vi "General wait for movement to stop.vi"(0 "System no.":i32=1, 2 "Axes to wait for":string[](array[string]), 3 "All axes?":bool=TRUE, 4 "Additional wait time, ms":u32, 5 "error in":errorcluster, 6 "Add. wait only?":bool, 7 "Polling cycle \ntime, ms":u32=10, 12 "Stop refnum":refnum<vi>) -> (14 "Stopped":bool, 19 "error out":errorcluster)   [LabVIEW 2026]
doc: "This VI waits for the specified axes to stop. An additional wait time can be specified. The wait method depends on the system to command. PI_GCS2_Configuration_Setup.vi must be run before running this VI. If Add. wait only? is TRUE, VI waits the given Additional wait time only. Requires Wait for axes to stop.vi, #5.vi, STA?.vi, #5_old.vi, ONT?.vi and Wait for hexapod system axes to stop.vi to be present. VI does not time out, so when using as a sub-VI, use Stop refnum to stop VI from caller.\n\nAnalog: If VOL was commanded or velocity control mode (VCO) is OFF, Add. wait only? must be TRUE, otherwise FALSE.\nE-816: All axes? = FALSE. only one axis per command allowed.\nC-887, F-206, M-8X0: For GCS syntax version = GCS 1.0 (Check with CSV?.vi. If CSV?.vi is not supported, syntax version is GCS 1.0), VI will not wait for INI procedure to complete."
uses:
  Communication/Syntax.ctl
  GeneralCommands/Global2 (Array).vi
  AnalogControl/Global Analog.vi
  Communication/Global1.vi
panel:
  in  "Local stop":bool
  # "This vi waits for the specified axes to stop. An additional wait\ntime can be specified. The wait method depends on the system\nto command. If \"Add. wait only?\" is TRUE, VI waits the given \nadditional wait time only. \"XXX_Configuration_Setup.vi\" must be\nrun before running this vi."
  # "Wait for"
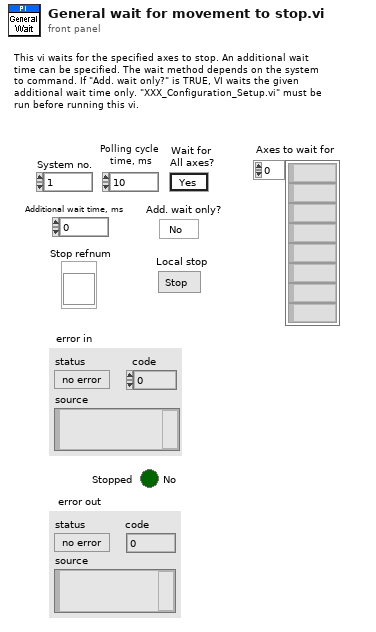
[diagram p1: front panel]
types:
  T1 = typedef "Controller names.ctl" = enum16{"None", "Analog", "C-702", "C-413", "C-414", "C-843", "C-843.PM", "C-844", "C-848", "C-865", "C-866", "C-867", "C-877", "C-880", "C-884", "C-885", "C-886", "C-887", "C-891", "E-135", "E-516", "E-517", "E-518", "E-709", "E-710", "E-712", "E-725", "E-727", "E-753", "E-754", "E-755", "E-761", "E-816", "E-861", "E-870", "E-871", "E-872", "E-873", "E-874", "F-206", "HydraPollux", "M-840", "M-850", "M-8X0", "Mercury", "Mercury_GCS", "PI_GCS2"}
  T2 = cluster{"Conn. axes":string[], "Controller name":T1}[]
  T3 = cluster{"Conn. axes":string[], "Controller name":T1}
  T4 = typedef "Syntax.ctl" = enum16{"GCS 1.0", "GCS 2.0", "GCS 3.0"}
  T5 = cluster{"Conversion factor":dbl[], "Velocity":dbl[], "Velocity control mode":bool, "AO.Resolution":dbl, "Lower voltage limit (V)":dbl, "Upper voltage limit (V)":dbl, "AO_WF_T (s)":dbl, "AI Sample Rate":dbl, "AI Samples/Channel":i32, "Hyperbit":bool, "Offset (V)":dbl[], "Hyperbit StayOnPos":bool, "Gain (V)":dbl[], "Bit rate (Hz)":dbl, "PWM rate (Hz)":dbl, "HyperBit Password":string, "AO.MaxRate":dbl, "Conversion offset":dbl[]}[]
  T6 = cluster{"Conversion factor":dbl[], "Velocity":dbl[], "Velocity control mode":bool, "AO.Resolution":dbl, "Lower voltage limit (V)":dbl, "Upper voltage limit (V)":dbl, "AO_WF_T (s)":dbl, "AI Sample Rate":dbl, "AI Samples/Channel":i32, "Hyperbit":bool, "Offset (V)":dbl[], "Hyperbit StayOnPos":bool, "Gain (V)":dbl[], "Bit rate (Hz)":dbl, "PWM rate (Hz)":dbl, "HyperBit Password":string, "AO.MaxRate":dbl, "Conversion offset":dbl[]}
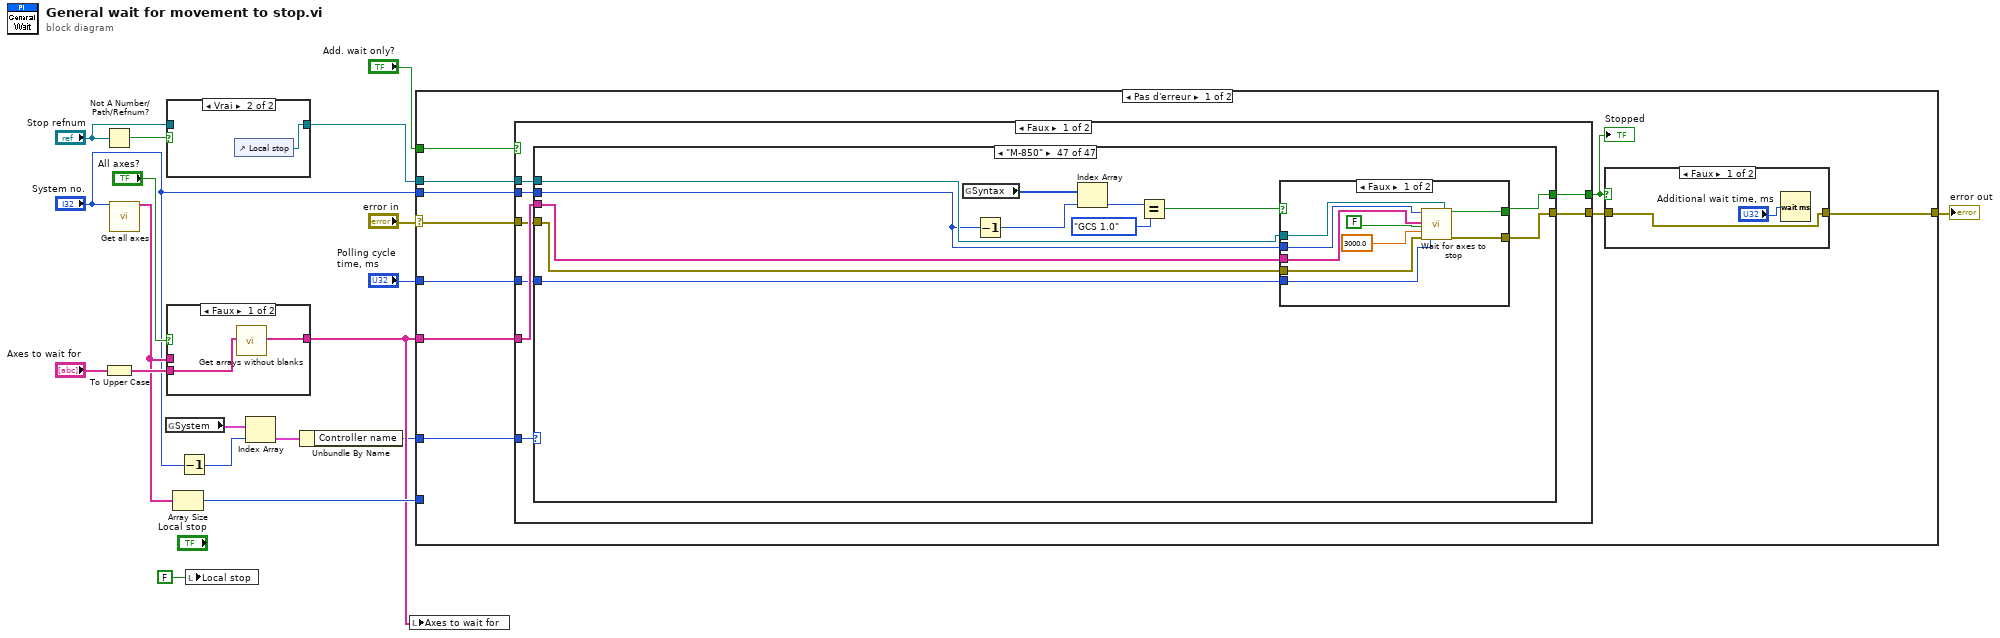
[diagram p0: block diagram]
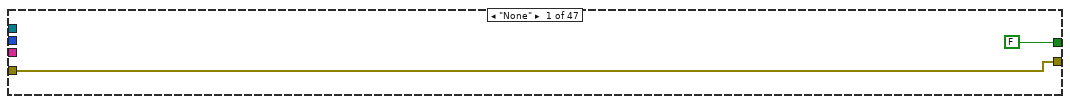
[diagram p4: hidden frame]
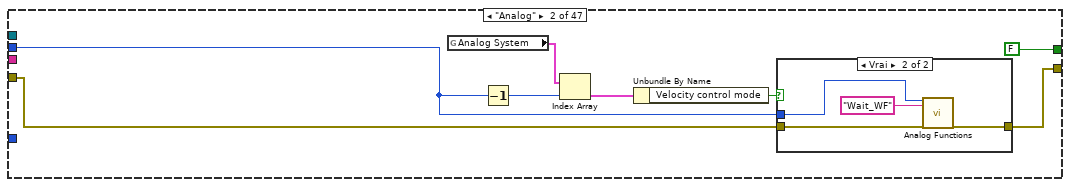
[diagram p5: hidden frame]
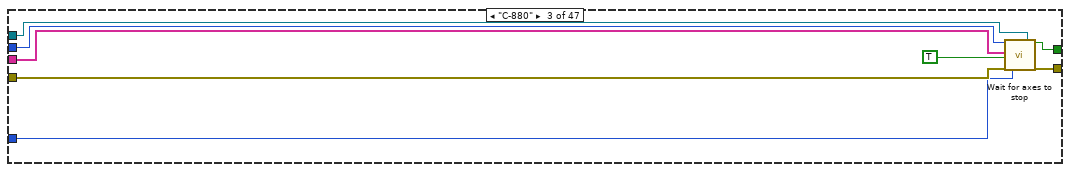
[diagram p7: hidden frame]
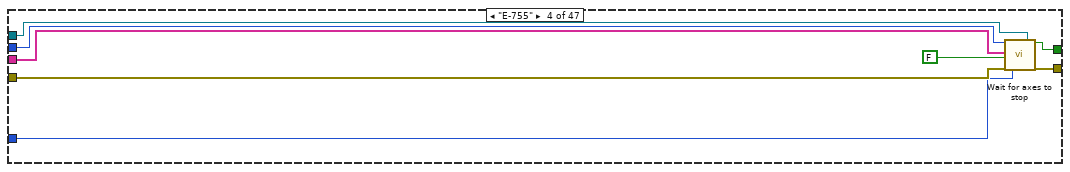
[diagram p8: hidden frame]
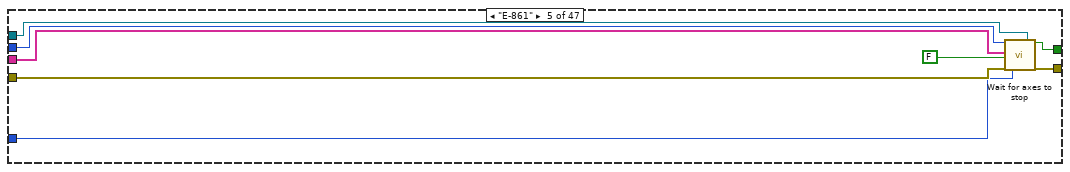
[diagram p9: hidden frame]
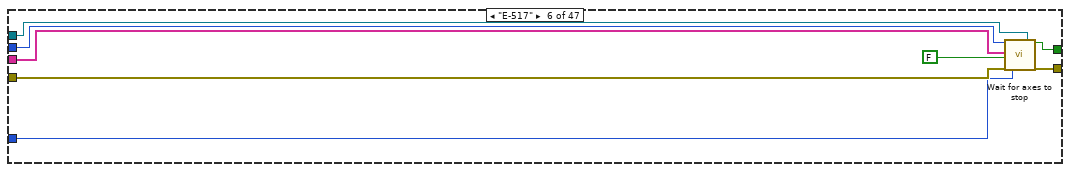
[diagram p10: hidden frame]
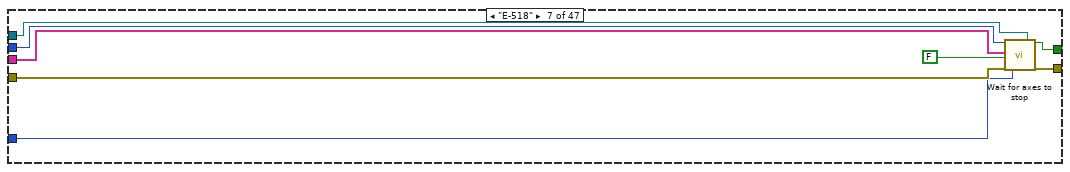
[diagram p11: hidden frame]
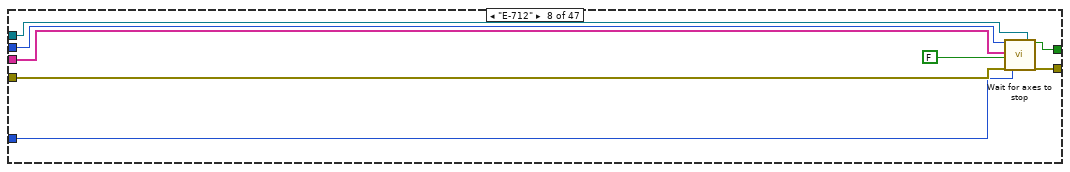
[diagram p12: hidden frame]
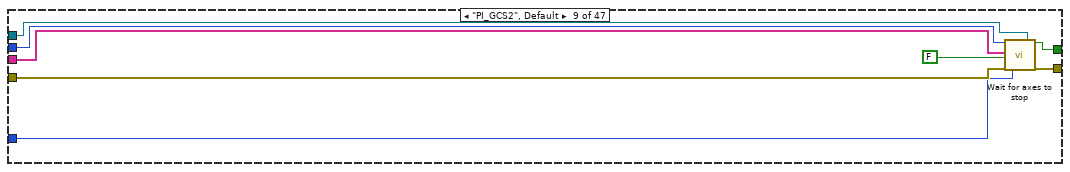
[diagram p13: hidden frame]
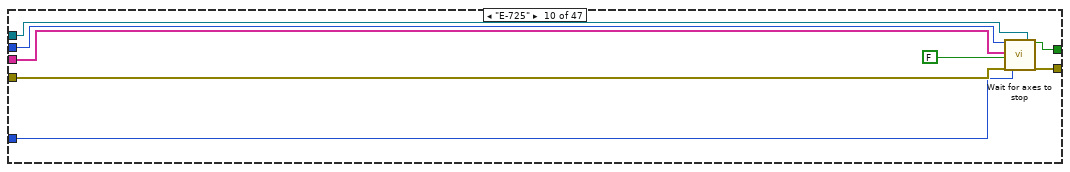
[diagram p14: hidden frame]
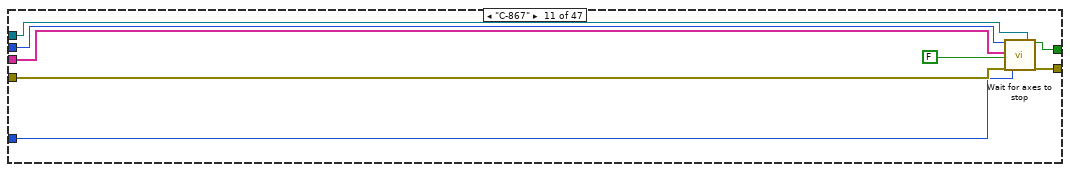
[diagram p15: hidden frame]
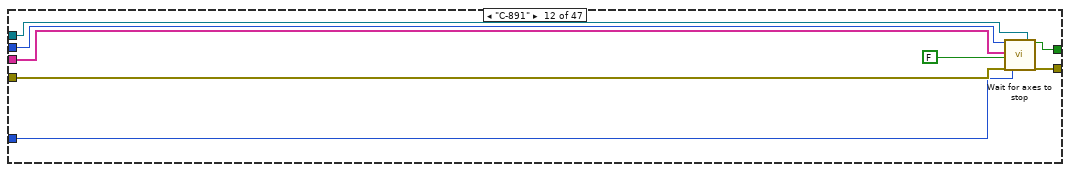
[diagram p16: hidden frame]
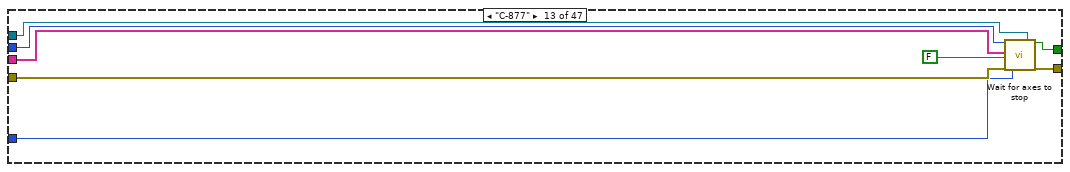
[diagram p17: hidden frame]
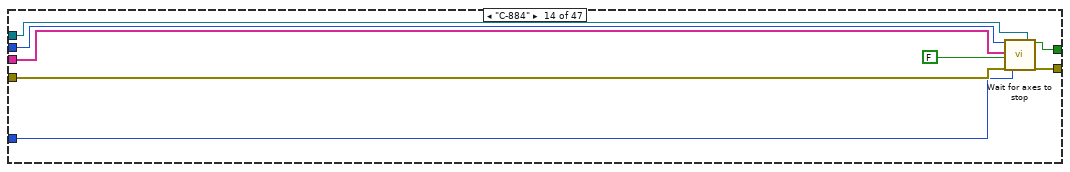
[diagram p18: hidden frame]
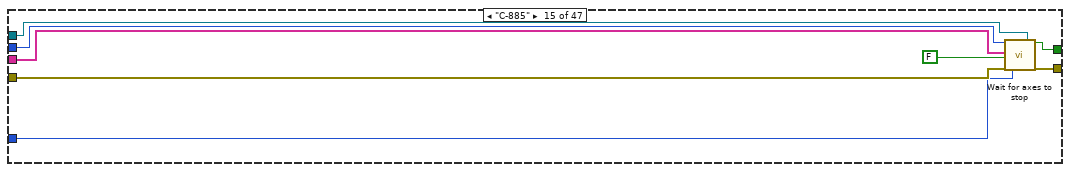
[diagram p19: hidden frame]
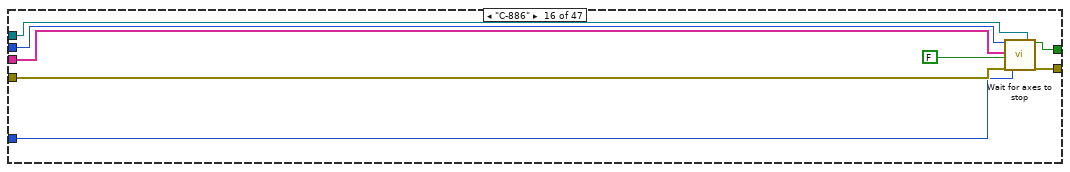
[diagram p20: hidden frame]
diagram:
  n1 = Not A Number/Path/Refnum?(number/path/refnum="Stop refnum") -> (NaN/Path/Refnum?=w11:bool)
  n2 = To Upper Case(1:"Axes to wait for") -> (0:w15:string[])
  n3 = call "Get all axes.vi"("System no."="System no.") -> ("Conn. Axes"=w6:string[])  [unwired: 18 out]
  n4 = global read "Global2 (Array).vi" "System"() -> (w8:T2)
  n5 = case shown="Vrai" w11 {
    tunnel: [w20 w21] -> w9
    tunnel: "Stop refnum" -> [w20 _]
    frame False {
    }
    frame True {
      n6 = control-ref of="Local stop"() -> (w21:refnum<vi>)
    }
  }
  n7 = case shown="Faux" "All axes?" {
    tunnel: [w22 w24] -> w14
    tunnel: w15 -> [w23 _]
    tunnel: w6 -> [_ w24]
    frame False {
      n8 = call "Get arrays without blanks.vi"("String array in"=w23) -> ("String array out"=w22:string[])  [unwired: 2 in, 16 out]
    }
    frame True {
    }
  }
  n9 = Array Size(array=w6) -> (size(s)=w18:i32)
  n10 = Decrement(x="System no.") -> (x-1=w4:i32)
  n11 = local write "Local stop"(FALSE ("Finished")) -> ()
  n12 = Index Array(array=w8, index=w4) -> (element=w7:T3)
  n13 = Unbundle By Name(w7) -> ("Controller name"=w3:T1)
  n14 = local write "Axes to wait for"(w14) -> ()
  n15 = case shown="Pas d'erreur" "error in" {
    selector: "error in" -> [w25 w600]
    tunnel: "System no." -> [w33 _]
    tunnel: w18 -> [_ _]
    tunnel: [w28 w600] -> w17
    tunnel: w3 -> [w34 _]
    tunnel: w14 -> [w32 _]
    tunnel: "Polling cycle \ntime, ms" -> [w31 _]
    tunnel: w9 -> [w30 _]
    tunnel: "Add. wait only?" -> [w26 _]
    frame No Error {
      n16 = case shown="Faux" w26 {
        tunnel: w34 -> [w42 _]
        tunnel: w33 -> [w41 _]
        tunnel: w32 -> [w40 _]
        tunnel: w25 -> [w39 w595]
        tunnel: w31 -> [w38 _]
        tunnel: w30 -> [w37 _]
        tunnel: [w36 w595] -> w29
        tunnel: [w35 FALSE ("Stopped")] -> w27
        frame False {
          n17 = case shown="\"M-850\"" w42 {
            tunnel: w41 -> [_ w47 w65 w73 w81 w89 w97 w105 w113 w121 w129 w137 w145 w153 w161 w169 w177 w185 w193 w201 w209 w217 w225 w233 w241 w249 w257 w265 w273 w281 w289 w297 w305 w313 w321 w329 w337 w345 w352 w379 w406 w433 w460 w484 w512 w540 w569]
            tunnel: w40 -> [_ _ w63 w71 w79 w87 w95 w103 w111 w119 w127 w135 w143 w151 w159 w167 w175 w183 w191 w199 w207 w215 w223 w231 w239 w247 w255 w263 w271 w279 w287 w295 w303 w311 w319 w327 w335 w343 w351 w378 w405 w432 w459 w494 w522 w550 w578]
            tunnel: [w44 w50 w59 w67 w75 w83 w91 w99 w107 w115 w123 w131 w139 w147 w155 w163 w171 w179 w187 w195 w203 w211 w219 w227 w235 w243 w251 w259 w267 w275 w283 w291 w299 w307 w315 w323 w331 w339 w349 w376 w403 w430 w458 w492 w520 w548 w576] -> w36
            tunnel: w39 -> [w44 w51 w62 w70 w78 w86 w94 w102 w110 w118 w126 w134 w142 w150 w158 w166 w174 w182 w190 w198 w206 w214 w222 w230 w238 w246 w254 w262 w270 w278 w286 w294 w302 w310 w318 w326 w334 w342 w350 w377 w404 w431 w455 w493 w521 w549 w577]
            tunnel: w38 -> [_ _ w61 w69 w77 w85 w93 w101 w109 w117 w125 w133 w141 w149 w157 w165 w173 w181 w189 w197 w205 w213 w221 w229 w237 w245 w253 w261 w269 w277 w285 w293 w301 w309 w317 w325 w333 w341 w346 w373 w400 w427 _ w483 w511 w539 w568]
            tunnel: w37 -> [_ _ w60 w68 w76 w84 w92 w100 w108 w116 w124 w132 w140 w148 w156 w164 w172 w180 w188 w196 w204 w212 w220 w228 w236 w244 w252 w260 w268 w276 w284 w292 w300 w308 w316 w324 w332 w340 w348 w375 w402 w429 w457 w491 w519 w547 w575]
            tunnel: [FALSE ("Stopped") FALSE ("Stopped") w58 w66 w74 w82 w90 w98 w106 w114 w122 w130 w138 w146 w154 w162 w170 w178 w186 w194 w202 w210 w218 w226 w234 w242 w250 w258 w266 w274 w282 w290 w298 w306 w314 w322 w330 w338 w347 w374 w401 w428 w456 w490 w518 w546 w574] -> w35
            frame "None" {
            }
            frame "Analog" {
              n18 = global read "Global Analog.vi" "Analog System"() -> (w49:T5)
              n19 = Decrement(x=w47) -> (x-1=w48:i32)
              n20 = Index Array(array=w49, index=w48) -> (element=w46:T6)
              n21 = Unbundle By Name(w46) -> ("Velocity control mode"=w45:bool)
              n22 = case shown="Vrai" w45 {
                tunnel: w47 -> [_ w57]
                tunnel: w51 -> [w53 w55]
                tunnel: [w53 w54] -> w50
                frame False {
                }
                frame True {
                  n23 = call "Analog Functions.vi"("System no."=w57, "String to send"="Wait_WF", "error in"=w55) -> ("error out"=w54:errorcluster)  [unwired: 4 in, 12 out]
                }
              }
            }
            frame "C-880" {
              n24 = call "Wait for axes to stop.vi"("System no."=w65, "Axes to wait for"=w63, "With status bit polling?"=TRUE, "error in"=w62, "Polling cycle time, ms"=w61, "Stop refnum"=w60) -> ("Stopped"=w58:bool, "error out"=w59:errorcluster)  [unwired: 1 in, 11 out]
            }
            frame "E-755" {
              n25 = call "Wait for axes to stop.vi"("System no."=w73, "Axes to wait for"=w71, "With status bit polling?"=FALSE, "error in"=w70, "Polling cycle time, ms"=w69, "Stop refnum"=w68) -> ("Stopped"=w66:bool, "error out"=w67:errorcluster)  [unwired: 1 in, 11 out]
            }
            frame "E-861" {
              n26 = call "Wait for axes to stop.vi"("System no."=w81, "Axes to wait for"=w79, "With status bit polling?"=FALSE, "error in"=w78, "Polling cycle time, ms"=w77, "Stop refnum"=w76) -> ("Stopped"=w74:bool, "error out"=w75:errorcluster)  [unwired: 1 in, 11 out]
            }
            frame "E-517" {
              n27 = call "Wait for axes to stop.vi"("System no."=w89, "Axes to wait for"=w87, "With status bit polling?"=FALSE, "error in"=w86, "Polling cycle time, ms"=w85, "Stop refnum"=w84) -> ("Stopped"=w82:bool, "error out"=w83:errorcluster)  [unwired: 1 in, 11 out]
            }
            frame "E-518" {
              n28 = call "Wait for axes to stop.vi"("System no."=w97, "Axes to wait for"=w95, "With status bit polling?"=FALSE, "error in"=w94, "Polling cycle time, ms"=w93, "Stop refnum"=w92) -> ("Stopped"=w90:bool, "error out"=w91:errorcluster)  [unwired: 1 in, 11 out]
            }
            frame "E-712" {
              n29 = call "Wait for axes to stop.vi"("System no."=w105, "Axes to wait for"=w103, "With status bit polling?"=FALSE, "error in"=w102, "Polling cycle time, ms"=w101, "Stop refnum"=w100) -> ("Stopped"=w98:bool, "error out"=w99:errorcluster)  [unwired: 1 in, 11 out]
            }
            frame "PI_GCS2", Default {
              n30 = call "Wait for axes to stop.vi"("System no."=w113, "Axes to wait for"=w111, "With status bit polling?"=FALSE, "error in"=w110, "Polling cycle time, ms"=w109, "Stop refnum"=w108) -> ("Stopped"=w106:bool, "error out"=w107:errorcluster)  [unwired: 1 in, 11 out]
            }
            frame "E-725" {
              n31 = call "Wait for axes to stop.vi"("System no."=w121, "Axes to wait for"=w119, "With status bit polling?"=FALSE, "error in"=w118, "Polling cycle time, ms"=w117, "Stop refnum"=w116) -> ("Stopped"=w114:bool, "error out"=w115:errorcluster)  [unwired: 1 in, 11 out]
            }
            frame "C-867" {
              n32 = call "Wait for axes to stop.vi"("System no."=w129, "Axes to wait for"=w127, "With status bit polling?"=FALSE, "error in"=w126, "Polling cycle time, ms"=w125, "Stop refnum"=w124) -> ("Stopped"=w122:bool, "error out"=w123:errorcluster)  [unwired: 1 in, 11 out]
            }
            frame "C-891" {
              n33 = call "Wait for axes to stop.vi"("System no."=w137, "Axes to wait for"=w135, "With status bit polling?"=FALSE, "error in"=w134, "Polling cycle time, ms"=w133, "Stop refnum"=w132) -> ("Stopped"=w130:bool, "error out"=w131:errorcluster)  [unwired: 1 in, 11 out]
            }
            frame "C-877" {
              n34 = call "Wait for axes to stop.vi"("System no."=w145, "Axes to wait for"=w143, "With status bit polling?"=FALSE, "error in"=w142, "Polling cycle time, ms"=w141, "Stop refnum"=w140) -> ("Stopped"=w138:bool, "error out"=w139:errorcluster)  [unwired: 1 in, 11 out]
            }
            frame "C-884" {
              n35 = call "Wait for axes to stop.vi"("System no."=w153, "Axes to wait for"=w151, "With status bit polling?"=FALSE, "error in"=w150, "Polling cycle time, ms"=w149, "Stop refnum"=w148) -> ("Stopped"=w146:bool, "error out"=w147:errorcluster)  [unwired: 1 in, 11 out]
            }
            frame "C-885" {
              n36 = call "Wait for axes to stop.vi"("System no."=w161, "Axes to wait for"=w159, "With status bit polling?"=FALSE, "error in"=w158, "Polling cycle time, ms"=w157, "Stop refnum"=w156) -> ("Stopped"=w154:bool, "error out"=w155:errorcluster)  [unwired: 1 in, 11 out]
            }
            frame "C-886" {
              n37 = call "Wait for axes to stop.vi"("System no."=w169, "Axes to wait for"=w167, "With status bit polling?"=FALSE, "error in"=w166, "Polling cycle time, ms"=w165, "Stop refnum"=w164) -> ("Stopped"=w162:bool, "error out"=w163:errorcluster)  [unwired: 1 in, 11 out]
            }
            frame "C-887" {
              n38 = call "Wait for axes to stop.vi"("System no."=w177, "Axes to wait for"=w175, "With status bit polling?"=FALSE, "error in"=w174, "Polling cycle time, ms"=w173, "Stop refnum"=w172) -> ("Stopped"=w170:bool, "error out"=w171:errorcluster)  [unwired: 1 in, 11 out]
            }
            frame "E-871" {
              n39 = call "Wait for axes to stop.vi"("System no."=w185, "Axes to wait for"=w183, "With status bit polling?"=FALSE, "error in"=w182, "Polling cycle time, ms"=w181, "Stop refnum"=w180) -> ("Stopped"=w178:bool, "error out"=w179:errorcluster)  [unwired: 1 in, 11 out]
            }
            frame "E-872" {
              n40 = call "Wait for axes to stop.vi"("System no."=w193, "Axes to wait for"=w191, "With status bit polling?"=FALSE, "error in"=w190, "Polling cycle time, ms"=w189, "Stop refnum"=w188) -> ("Stopped"=w186:bool, "error out"=w187:errorcluster)  [unwired: 1 in, 11 out]
            }
            frame "E-135" {
              n41 = call "Wait for axes to stop.vi"("System no."=w201, "Axes to wait for"=w199, "With status bit polling?"=FALSE, "error in"=w198, "Polling cycle time, ms"=w197, "Stop refnum"=w196) -> ("Stopped"=w194:bool, "error out"=w195:errorcluster)  [unwired: 1 in, 11 out]
            }
            frame "E-873" {
              n42 = call "Wait for axes to stop.vi"("System no."=w209, "Axes to wait for"=w207, "With status bit polling?"=FALSE, "error in"=w206, "Polling cycle time, ms"=w205, "Stop refnum"=w204) -> ("Stopped"=w202:bool, "error out"=w203:errorcluster)  [unwired: 1 in, 11 out]
            }
            frame "E-874" {
              n43 = call "Wait for axes to stop.vi"("System no."=w217, "Axes to wait for"=w215, "With status bit polling?"=FALSE, "error in"=w214, "Polling cycle time, ms"=w213, "Stop refnum"=w212) -> ("Stopped"=w210:bool, "error out"=w211:errorcluster)  [unwired: 1 in, 11 out]
            }
            frame "C-413" {
              n44 = call "Wait for axes to stop.vi"("System no."=w225, "Axes to wait for"=w223, "With status bit polling?"=FALSE, "error in"=w222, "Polling cycle time, ms"=w221, "Stop refnum"=w220) -> ("Stopped"=w218:bool, "error out"=w219:errorcluster)  [unwired: 1 in, 11 out]
            }
            frame "C-414" {
              n45 = call "Wait for axes to stop.vi"("System no."=w233, "Axes to wait for"=w231, "With status bit polling?"=FALSE, "error in"=w230, "Polling cycle time, ms"=w229, "Stop refnum"=w228) -> ("Stopped"=w226:bool, "error out"=w227:errorcluster)  [unwired: 1 in, 11 out]
            }
            frame "E-870" {
              n46 = call "Wait for axes to stop.vi"("System no."=w241, "Axes to wait for"=w239, "With status bit polling?"=FALSE, "error in"=w238, "Polling cycle time, ms"=w237, "Stop refnum"=w236) -> ("Stopped"=w234:bool, "error out"=w235:errorcluster)  [unwired: 1 in, 11 out]
            }
            frame "HydraPollux" {
              n47 = call "Wait for axes to stop.vi"("System no."=w249, "Axes to wait for"=w247, "With status bit polling?"=FALSE, "error in"=w246, "Polling cycle time, ms"=w245, "Stop refnum"=w244) -> ("Stopped"=w242:bool, "error out"=w243:errorcluster)  [unwired: 1 in, 11 out]
            }
            frame "Mercury_GCS" {
              n48 = call "Wait for axes to stop.vi"("System no."=w257, "Axes to wait for"=w255, "With status bit polling?"=FALSE, "error in"=w254, "Polling cycle time, ms"=w253, "Stop refnum"=w252) -> ("Stopped"=w250:bool, "error out"=w251:errorcluster)  [unwired: 1 in, 11 out]
            }
            frame "E-753" {
              n49 = call "Wait for axes to stop.vi"("System no."=w265, "Axes to wait for"=w263, "With status bit polling?"=FALSE, "error in"=w262, "Polling cycle time, ms"=w261, "Stop refnum"=w260) -> ("Stopped"=w258:bool, "error out"=w259:errorcluster)  [unwired: 1 in, 11 out]
            }
            frame "E-727" {
              n50 = call "Wait for axes to stop.vi"("System no."=w273, "Axes to wait for"=w271, "With status bit polling?"=FALSE, "error in"=w270, "Polling cycle time, ms"=w269, "Stop refnum"=w268) -> ("Stopped"=w266:bool, "error out"=w267:errorcluster)  [unwired: 1 in, 11 out]
            }
            frame "E-754" {
              n51 = call "Wait for axes to stop.vi"("System no."=w281, "Axes to wait for"=w279, "With status bit polling?"=FALSE, "error in"=w278, "Polling cycle time, ms"=w277, "Stop refnum"=w276) -> ("Stopped"=w274:bool, "error out"=w275:errorcluster)  [unwired: 1 in, 11 out]
            }
            frame "E-709" {
              n52 = call "Wait for axes to stop.vi"("System no."=w289, "Axes to wait for"=w287, "With status bit polling?"=FALSE, "error in"=w286, "Polling cycle time, ms"=w285, "Stop refnum"=w284) -> ("Stopped"=w282:bool, "error out"=w283:errorcluster)  [unwired: 1 in, 11 out]
            }
            frame "C-702" {
              n53 = call "Wait for axes to stop.vi"("System no."=w297, "Axes to wait for"=w295, "With status bit polling?"=FALSE, "error in"=w294, "Polling cycle time, ms"=w293, "Stop refnum"=w292) -> ("Stopped"=w290:bool, "error out"=w291:errorcluster)  [unwired: 1 in, 11 out]
            }
            frame "C-848" {
              n54 = call "Wait for axes to stop.vi"("System no."=w305, "Axes to wait for"=w303, "With status bit polling?"=TRUE, "error in"=w302, "Polling cycle time, ms"=w301, "Stop refnum"=w300) -> ("Stopped"=w298:bool, "error out"=w299:errorcluster)  [unwired: 1 in, 11 out]
            }
            frame "C-843" {
              n55 = call "Wait for axes to stop.vi"("System no."=w313, "Axes to wait for"=w311, "With status bit polling?"=FALSE, "error in"=w310, "Polling cycle time, ms"=w309, "Stop refnum"=w308) -> ("Stopped"=w306:bool, "error out"=w307:errorcluster)  [unwired: 1 in, 11 out]
            }
            frame "C-843.PM" {
              n56 = call "Wait for axes to stop.vi"("System no."=w321, "Axes to wait for"=w319, "With status bit polling?"=FALSE, "error in"=w318, "Polling cycle time, ms"=w317, "Stop refnum"=w316) -> ("Stopped"=w314:bool, "error out"=w315:errorcluster)  [unwired: 1 in, 11 out]
            }
            frame "C-865" {
              n57 = call "Wait for axes to stop.vi"("System no."=w329, "Axes to wait for"=w327, "With status bit polling?"=FALSE, "error in"=w326, "Polling cycle time, ms"=w325, "Stop refnum"=w324) -> ("Stopped"=w322:bool, "error out"=w323:errorcluster)  [unwired: 1 in, 11 out]
            }
            frame "C-866" {
              n58 = call "Wait for axes to stop.vi"("System no."=w337, "Axes to wait for"=w335, "With status bit polling?"=FALSE, "error in"=w334, "Polling cycle time, ms"=w333, "Stop refnum"=w332) -> ("Stopped"=w330:bool, "error out"=w331:errorcluster)  [unwired: 1 in, 11 out]
            }
            frame "C-844" {
              n59 = call "Wait for axes to stop.vi"("System no."=w345, "Axes to wait for"=w343, "With status bit polling?"=FALSE, "error in"=w342, "Polling cycle time, ms"=w341, "Stop refnum"=w340) -> ("Stopped"=w338:bool, "error out"=w339:errorcluster)  [unwired: 1 in, 11 out]
            }
            frame "E-516" {
              n60 = while {
                tunnel: [w354] -> w347
                tunnel: w348 -> [w355]
                shift-left: w350 -> [w363]
                shift-right: [w356] -> w349
                tunnel: w351 -> [w365]
                tunnel: w352 -> [w366]
                tunnel: w346 -> [w353]
                stop <- w359 continue-if-true
                n61 = property class="Bool (strict)"(reference=w355) -> ("Value"=w354:bool)  [unwired: 1 in, 2 out]
                n62 = Wait Until Next ms Multiple(millisecond multiple=w353) -> ()  [unwired: 1 out]
                n63 = call "qONT.vi"("System no."=w366, "Axes to query"=w365, "All axes?"=FALSE, "error in"=w363) -> ("Axis on target?"=w362:bool[], "error out"=w357:errorcluster)  [unwired: 1 in, 13 out]
                n64 = Unbundle By Name(w357) -> ("status"=w361:bool)
                n65 = case shown="Vrai" w354 {
                  tunnel: w357 -> [w367 w368]
                  tunnel: [w367 w369] -> w356
                  frame False {
                  }
                  frame True {
                    n66 = Bundle By Name(cluster=w368, "status"=FALSE, "code"=0, "source"="Warning: General wait for\nmovement to stop was stopped.") -> (w369:errorcluster)
                  }
                }
                n67 = And Array Elements(Boolean array=w362) -> (logical AND=w358:bool)
                n68 = Compound Arithmetic op=OR(w358, w361, w354) -> (w360:bool)
                n69 = Not(x=w360) -> (.not. x?=w359:bool)
              }
            }
            frame "E-761" {
              n70 = while {
                tunnel: [w381] -> w374
                tunnel: w375 -> [w382]
                shift-left: w377 -> [w390]
                shift-right: [w383] -> w376
                tunnel: w378 -> [w392]
                tunnel: w379 -> [w393]
                tunnel: w373 -> [w380]
                stop <- w386 continue-if-true
                n71 = property class="Bool (strict)"(reference=w382) -> ("Value"=w381:bool)  [unwired: 1 in, 2 out]
                n72 = Wait Until Next ms Multiple(millisecond multiple=w380) -> ()  [unwired: 1 out]
                n73 = call "qONT.vi"("System no."=w393, "Axes to query"=w392, "All axes?"=FALSE, "error in"=w390) -> ("Axis on target?"=w389:bool[], "error out"=w384:errorcluster)  [unwired: 1 in, 13 out]
                n74 = Unbundle By Name(w384) -> ("status"=w388:bool)
                n75 = case shown="Vrai" w381 {
                  tunnel: w384 -> [w394 w395]
                  tunnel: [w394 w396] -> w383
                  frame False {
                  }
                  frame True {
                    n76 = Bundle By Name(cluster=w395, "status"=FALSE, "code"=0, "source"="Warning: General wait for\nmovement to stop was stopped.") -> (w396:errorcluster)
                  }
                }
                n77 = And Array Elements(Boolean array=w389) -> (logical AND=w385:bool)
                n78 = Compound Arithmetic op=OR(w385, w388, w381) -> (w387:bool)
                n79 = Not(x=w387) -> (.not. x?=w386:bool)
              }
            }
            frame "E-710" {
              n80 = while {
                tunnel: [w408] -> w401
                tunnel: w402 -> [w409]
                shift-left: w404 -> [w417]
                shift-right: [w410] -> w403
                tunnel: w405 -> [w419]
                tunnel: w406 -> [w420]
                tunnel: w400 -> [w407]
                stop <- w413 continue-if-true
                n81 = property class="Bool (strict)"(reference=w409) -> ("Value"=w408:bool)  [unwired: 1 in, 2 out]
                n82 = Wait Until Next ms Multiple(millisecond multiple=w407) -> ()  [unwired: 1 out]
                n83 = call "qONT.vi"("System no."=w420, "Axes to query"=w419, "All axes?"=FALSE, "error in"=w417) -> ("Axis on target?"=w416:bool[], "error out"=w411:errorcluster)  [unwired: 1 in, 13 out]
                n84 = Unbundle By Name(w411) -> ("status"=w415:bool)
                n85 = case shown="Vrai" w408 {
                  tunnel: w411 -> [w421 w422]
                  tunnel: [w421 w423] -> w410
                  frame False {
                  }
                  frame True {
                    n86 = Bundle By Name(cluster=w422, "status"=FALSE, "code"=0, "source"="Warning: General wait for\nmovement to stop was stopped.") -> (w423:errorcluster)
                  }
                }
                n87 = And Array Elements(Boolean array=w416) -> (logical AND=w412:bool)
                n88 = Compound Arithmetic op=OR(w412, w415, w408) -> (w414:bool)
                n89 = Not(x=w414) -> (.not. x?=w413:bool)
              }
            }
            frame "Mercury" {
              n90 = while {
                tunnel: [w435] -> w428
                tunnel: w429 -> [w436]
                shift-left: w431 -> [w444]
                shift-right: [w437] -> w430
                tunnel: w432 -> [w446]
                tunnel: w433 -> [w447]
                tunnel: w427 -> [w434]
                stop <- w440 continue-if-true
                n91 = property class="Bool (strict)"(reference=w436) -> ("Value"=w435:bool)  [unwired: 1 in, 2 out]
                n92 = Wait Until Next ms Multiple(millisecond multiple=w434) -> ()  [unwired: 1 out]
                n93 = call "qONT.vi"("System no."=w447, "Axes to query"=w446, "All axes?"=FALSE, "error in"=w444) -> ("Axis on target?"=w443:bool[], "error out"=w438:errorcluster)  [unwired: 1 in, 13 out]
                n94 = Unbundle By Name(w438) -> ("status"=w442:bool)
                n95 = case shown="Vrai" w435 {
                  tunnel: w438 -> [w448 w449]
                  tunnel: [w448 w450] -> w437
                  frame False {
                  }
                  frame True {
                    n96 = Bundle By Name(cluster=w449, "status"=FALSE, "code"=0, "source"="Warning: General wait for\nmovement to stop was stopped.") -> (w450:errorcluster)
                  }
                }
                n97 = And Array Elements(Boolean array=w443) -> (logical AND=w439:bool)
                n98 = Compound Arithmetic op=OR(w439, w442, w435) -> (w441:bool)
                n99 = Not(x=w441) -> (.not. x?=w440:bool)
              }
            }
            frame "E-816" {
              n100 = stacked-sequence {
                tunnel: w455 -> [w461]
                tunnel: [w461] -> w454
                frame #0 {
                  n101 = Wait (ms)(milliseconds to wait=u32 20) -> ()  [unwired: 1 out]
                }
              }
              n102 = while {
                tunnel: [w465] -> w456
                tunnel: w457 -> [w464]
                shift-left: w454 -> [w474]
                shift-right: [w466] -> w458
                tunnel: w459 -> [w475]
                tunnel: w460 -> [w476]
                stop <- w470 continue-if-true
                n103 = property class="Bool (strict)"(reference=w464) -> ("Value"=w465:bool)  [unwired: 1 in, 2 out]
                n104 = call "qONT.vi"("System no."=w476, "Axes to query"=w475, "All axes?"=FALSE, "error in"=w474) -> ("Axis on target?"=w473:bool[], "error out"=w467:errorcluster)  [unwired: 4 in, 10 out]
                n105 = Unbundle By Name(w467) -> ("status"=w472:bool)
                n106 = case shown="Vrai" w465 {
                  tunnel: w467 -> [w477 w478]
                  tunnel: [w477 w479] -> w466
                  frame False {
                  }
                  frame True {
                    n107 = Bundle By Name(cluster=w478, "status"=FALSE, "code"=0, "source"="Warning: General wait for\nmovement to stop was stopped.") -> (w479:errorcluster)
                  }
                }
                n108 = And Array Elements(Boolean array=w473) -> (logical AND=w469:bool)
                n109 = Compound Arithmetic op=OR(w469, w472, w465) -> (w471:bool)
                n110 = Not(x=w471) -> (.not. x?=w470:bool)
                n111 = Wait Until Next ms Multiple(millisecond multiple=u32 50) -> ()  [unwired: 1 out]
              }
            }
            frame "M-8X0" {
              n112 = global read "Global1.vi" "Syntax"() -> (w486:T4[])
              n113 = Decrement(x=w484) -> (x-1=w487:i32)
              n114 = Index Array(array=w486, index=w487) -> (element=w488:T4)
              n115 = Equal?(x=w488, y=enum16{"GCS 1.0", "GCS 2.0"}."GCS 1.0") -> (x = y?=w485:bool)
              n116 = case shown="Faux" w485 {
                tunnel: w484 -> [w499 w510]
                tunnel: w494 -> [w498 w509]
                tunnel: w493 -> [w503 w508]
                tunnel: [w502 w506] -> w492
                tunnel: w491 -> [w500 w505]
                tunnel: [w501 w504] -> w490
                tunnel: w483 -> [w495 _]
                frame False {
                  n117 = call "Wait for axes to stop.vi"("System no."=w499, "Axes to wait for"=w498, "With status bit polling?"=FALSE, "Timeout (s)"=3000.0, "error in"=w503, "Polling cycle time, ms"=w495, "Stop refnum"=w500) -> ("Stopped"=w501:bool, "error out"=w502:errorcluster)  [unwired: 11 out]
                }
                frame True {
                  n118 = call "Wait for hexapod system axes to stop.vi"("System no."=w510, "Axes to wait for"=w509, "All axes?"=FALSE, "error in"=w508, "Stop refnum"=w505) -> ("Stopped"=w504:bool, "error out"=w506:errorcluster)  [unwired: 13 out]
                }
              }
            }
            frame "F-206" {
              n119 = global read "Global1.vi" "Syntax"() -> (w514:T4[])
              n120 = Decrement(x=w512) -> (x-1=w515:i32)
              n121 = Index Array(array=w514, index=w515) -> (element=w516:T4)
              n122 = Equal?(x=w516, y=enum16{"GCS 1.0", "GCS 2.0"}."GCS 1.0") -> (x = y?=w513:bool)
              n123 = case shown="Faux" w513 {
                tunnel: w512 -> [w527 w538]
                tunnel: w522 -> [w526 w537]
                tunnel: w521 -> [w531 w536]
                tunnel: [w530 w534] -> w520
                tunnel: w519 -> [w528 w533]
                tunnel: [w529 w532] -> w518
                tunnel: w511 -> [w523 _]
                frame False {
                  n124 = call "Wait for axes to stop.vi"("System no."=w527, "Axes to wait for"=w526, "With status bit polling?"=FALSE, "Timeout (s)"=3000.0, "error in"=w531, "Polling cycle time, ms"=w523, "Stop refnum"=w528) -> ("Stopped"=w529:bool, "error out"=w530:errorcluster)  [unwired: 11 out]
                }
                frame True {
                  n125 = call "Wait for hexapod system axes to stop.vi"("System no."=w538, "Axes to wait for"=w537, "All axes?"=FALSE, "error in"=w536, "Stop refnum"=w533) -> ("Stopped"=w532:bool, "error out"=w534:errorcluster)  [unwired: 13 out]
                }
              }
            }
            frame "M-840" {
              n126 = global read "Global1.vi" "Syntax"() -> (w542:T4[])
              n127 = Decrement(x=w540) -> (x-1=w543:i32)
              n128 = Index Array(array=w542, index=w543) -> (element=w544:T4)
              n129 = Equal?(x=w544, y=enum16{"GCS 1.0", "GCS 2.0"}."GCS 1.0") -> (x = y?=w541:bool)
              n130 = case shown="Faux" w541 {
                tunnel: w540 -> [w555 w566]
                tunnel: w550 -> [w554 w565]
                tunnel: w549 -> [w559 w564]
                tunnel: [w558 w562] -> w548
                tunnel: w547 -> [w556 w561]
                tunnel: [w557 w560] -> w546
                tunnel: w539 -> [w551 _]
                frame False {
                  n131 = call "Wait for axes to stop.vi"("System no."=w555, "Axes to wait for"=w554, "With status bit polling?"=FALSE, "Timeout (s)"=3000.0, "error in"=w559, "Polling cycle time, ms"=w551, "Stop refnum"=w556) -> ("Stopped"=w557:bool, "error out"=w558:errorcluster)  [unwired: 11 out]
                }
                frame True {
                  n132 = call "Wait for hexapod system axes to stop.vi"("System no."=w566, "Axes to wait for"=w565, "All axes?"=FALSE, "error in"=w564, "Stop refnum"=w561) -> ("Stopped"=w560:bool, "error out"=w562:errorcluster)  [unwired: 13 out]
                }
              }
            }
            frame "M-850" {
              n133 = global read "Global1.vi" "Syntax"() -> (w571:T4[])
              n134 = Decrement(x=w569) -> (x-1=w572:i32)
              n135 = Index Array(array=w571, index=w572) -> (element=w573:T4)
              n136 = Equal?(x=w573, y=Syntax."GCS 1.0") -> (x = y?=w570:bool)
              n137 = case shown="Faux" w570 {
                tunnel: w569 -> [w583 w594]
                tunnel: w578 -> [w582 w593]
                tunnel: w577 -> [w587 w592]
                tunnel: [w586 w590] -> w576
                tunnel: w575 -> [w584 w589]
                tunnel: [w585 w588] -> w574
                tunnel: w568 -> [w579 _]
                frame False {
                  n138 = call "Wait for axes to stop.vi"("System no."=w583, "Axes to wait for"=w582, "With status bit polling?"=FALSE, "Timeout (s)"=3000.0, "error in"=w587, "Polling cycle time, ms"=w579, "Stop refnum"=w584) -> ("Stopped"=w585:bool, "error out"=w586:errorcluster)  [unwired: 11 out]
                }
                frame True {
                  n139 = call "Wait for hexapod system axes to stop.vi"("System no."=w594, "Axes to wait for"=w593, "All axes?"=FALSE, "error in"=w592, "Stop refnum"=w589) -> ("Stopped"=w588:bool, "error out"=w590:errorcluster)  [unwired: 13 out]
                }
              }
            }
          }
        }
        frame True {
        }
      }
      "Stopped" <- w27
      n140 = case shown="Faux" w27 {
        tunnel: w29 -> [w597 w599]
        tunnel: [w597 w599] -> w28
        frame False {
          n141 = Wait (ms)(milliseconds to wait="Additional wait time, ms") -> ()  [unwired: 1 out]
        }
        frame True {
        }
      }
    }
    frame Error {
    }
  }
  "error out" <- w17
